vi "Complete 1 Round.vi"(0 "Elves in":set{T1}(c389), 1 "Movement Proposal Rules":T2(array[cluster])) -> (2 "Elves out":set{T1}(c389))   [LabVIEW 2020, in "AoC 2022.lvlib"]
uses:
  AoC 2022.lvlib
  Day 15 - Beacon Exclusion Zone/private/Location.ctl
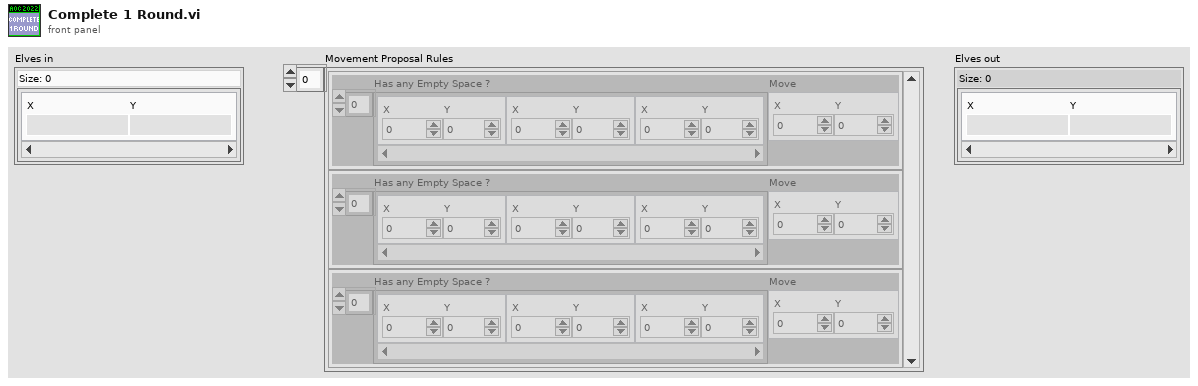
[diagram p1: front panel]
types:
  T1 = typedef "AoC 2022.lvlib/Location.ctl" = cluster{"X":i32, "Y":i32}
  T2 = cluster{"Has any Empty Space ?":T1[], "Move":T1}[]
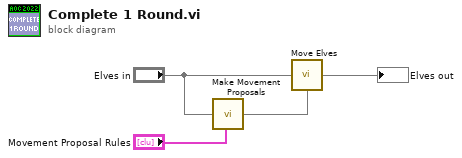
[diagram p0: block diagram]
diagram:
  n1 = call "Make Movement Proposals.vi"("Elves in"="Elves in", "Movement Proposal Rules"="Movement Proposal Rules") -> ("Elves' Movement Proposals"=w2:map{T1, T1})
  n2 = call "Move Elves.vi"("Elves in"="Elves in", "Elves' Movement Proposals"=w2) -> ("Elves out"=→"Elves out":set{T1})
